vi "Pfeiffer Vacuum Errors and Warnings.vi"(8 "error in (no error)":errorcluster, 9 "Position :":u16=1 min=1 max=10 step=1, 10 "Adress of unit":u16=1 min=1 max=999 step=1, 11 "VISA session in":refnum<visa-resource-name>) -> (0 "error out":errorcluster, 2 "Description of error":string, 3 "response (data)":string)   [LabVIEW 2016]
doc: "This VI is an example of how to use the Pfeiffer Vacuum subVIs programmatically. This VI first initializes the instrument, takes measurements, then closes the instrument."
uses:
  Pfeiffer Vacuum.lvlib
panel:
  # "Read error storage at"
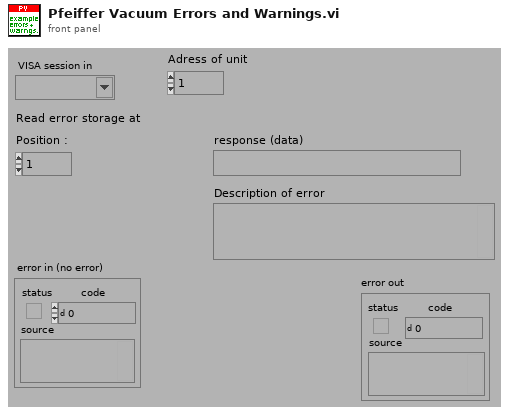
[diagram p1: front panel]
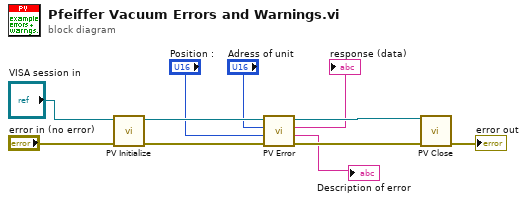
[diagram p0: block diagram]
diagram:
  n1 = call "PV Initialize.vi"("error in (no error)"="error in (no error)", "VISA session in"="VISA session in") -> ("error out"=w11:errorcluster, "VISA session out"=w9:refnum<visa-resource-name>)  [unwired: 8 in]
  n2 = call "PV Error.vi"("error in (no error)"=w11, "Position :"="Position :", "Adress of unit"="Adress of unit", "VISA session"=w9) -> ("error out"=w10:errorcluster, "Description of error"=→"Description of error":string, "response (data)"=→"response (data)":string, "dup VISA session"=w8:refnum<visa-resource-name>)  [unwired: 4 in]
  n3 = call "PV Close.vi"("VISA session"=w8, "error in (no error)"=w10) -> ("error out"=→"error out":errorcluster)  [unwired: 13 in]
